vi "Reset State.vi"(8 "error in (no error)":errorcluster, 11 "LoggingControl in":refnum<class "GroupLoggingControl.lvclass">) -> (0 "error out":errorcluster, 3 "LoggingControl out":refnum<class "GroupLoggingControl.lvclass">)   [LabVIEW 2020, in "VolatusGUIElements.lvlib" / "GroupLoggingControl.lvclass"]
uses:
  GroupLoggingControl.lvclass
  GroupLoggingControl.lvclass/GroupLoggingControl.ctl
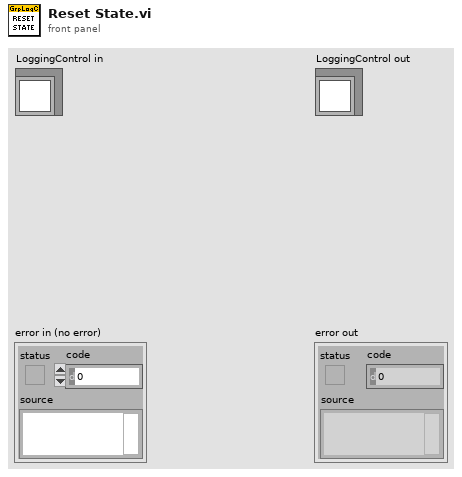
[diagram p1: front panel]
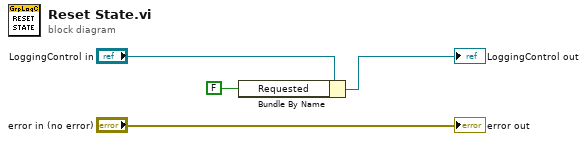
[diagram p0: block diagram]
diagram:
  n1 = Bundle By Name(cluster="LoggingControl in", "Requested"=FALSE ("State.Requested")) -> (→"LoggingControl out":refnum<class "GroupLoggingControl.lvclass">)
  "error out" <- "error in (no error)"
